vi "Timer.vi"(10 "RST":bool) -> (2 "time (Secs)":dbl)   [LabVIEW 2023]
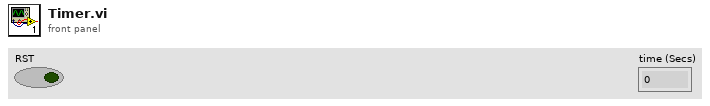
[diagram p1: front panel]
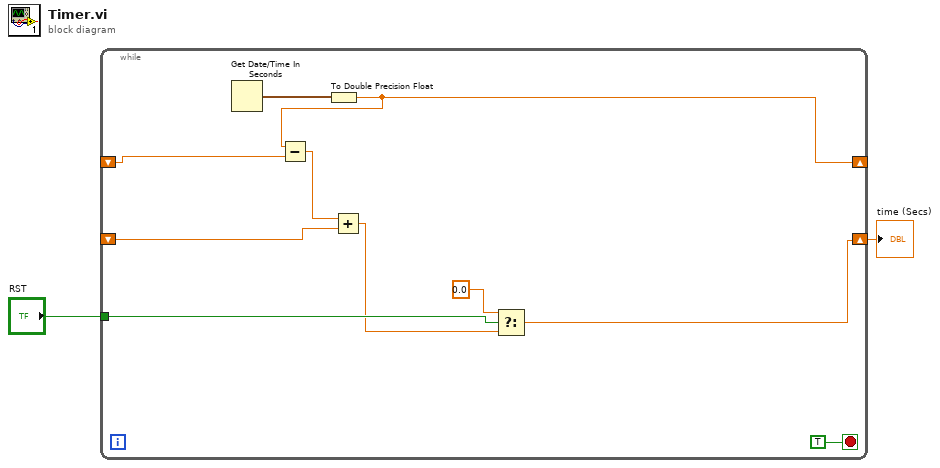
[diagram p0: block diagram]
diagram:
  n1 = while {
    shift-right: [w8] -> _
    shift-left: _ -> [w12]
    shift-right: [w3] -> w2
    shift-left: _ -> [w10]
    tunnel: "RST" -> [w6]
    stop <- TRUE stop-if-true
    n2 = Get Date/Time In Seconds() -> (seconds since 1Jan1904=w11:timestamp)
    n3 = To Double Precision Float(number=w11) -> (double precision float=w8:dbl)
    n4 = Subtract(x=w8, y=w12) -> (x-y=w9:dbl)
    n5 = Add(x=w9, y=w10) -> (x+y=w5:dbl)
    n6 = Select(t=0.0, s=w6, f=w5) -> (s? t:f=w3:dbl)
  }
  "time (Secs)" <- w2
